vi "Periodic Tasks.vi"(8 "error in":errorcluster) -> ()   [LabVIEW 2015]
doc: "This VI runs in parallel to other tasks. It can contain as many user-defined periodic loops as you need. These can carry out PID or other sorts of timed response."
uses:
  Controls/ShooterState.ctl
  <vilib>/Rock Robotics/WPI/CAN/TalonSRX/WPI_CANTalonSRX_APIControlMode.ctl
  <vilib>/Rock Robotics/WPI/CAN/TalonSRX/WPI_CANTalonSRX_APIFeedbackSelect.ctl
  <vilib>/Rock Robotics/WPI/Utilities/WPI_GetSetVariantRefNum.vi
  <vilib>/Rock Robotics/WPI/MotorControl/WPI_MotorControlOpenCANTalonSRX.vi
  <vilib>/Rock Robotics/Network Tables/NT Read Boolean.vi
  Robot Global Data.vi
  <vilib>/Rock Robotics/Network Tables/NT Write Boolean.vi
  <vilib>/Rock Robotics/Network Tables/NT Write Number.vi
  navX-MXP-LabVIEW/navX Library v2/navX Library v2.lvlib
panel:
  in  "High Shoot RPM":dbl=15000.0
  in  "Low Shoot RPM":dbl=5000.0
  in  "Intake Outtake RPM":dbl=2000.0
  in  "Shoot High":dbl(slide)=0.708955223880597 scale=0.0..1.0
  in  "Intake Outtake":dbl(slide)=0.208955223880597 scale=0.0..1.0
  in  "Shoot Low":dbl(slide)=0.43283582089552236 scale=0.0..1.0
  out "Actual Speed Chart":dbl(graph)
  out "Actual Speed":dbl(knob) scale=-20000.0..20000.0 scale format="%4d"
  in  "Test Speed":dbl(slide)=0.6712328767123288 scale=0.0..1.0
  in  "TEST Device #":u8=2
  in  "Throttle Ramp Rate (percent/s)":dbl=1.0
  out "Current Feedback":dbl(graph)
  in  "F":dbl(slide)=0.025 scale=0.0..1.0
  in  "D":dbl(slide)=13.3 scale=0.0..10.0
  in  "I":dbl(slide)=2.47 scale=0.0..5.0
  in  "P":dbl(slide)=0.1573 scale=0.0..20.0
  in  "Set Speed (RPM)":dbl(slide) scale=0.0..20000.0
  out "Shooter State":T1=enum."No Movement"
  in  "Outtake Button":i32=2
  in  "Low Shoot":i32=1
  in  "High Shoot Button":i32=3
  in  "Intake Button":i32
  in  "I":dbl=2.473
  in  "F":dbl=0.025
  in  "D":dbl=13.3
  in  "P":dbl=0.1573
  in  "Reverse Feedback Sensor":bool
  in  "Slave Device Number":u8=3
  in  "Encoder Codes Per Rev":u16=1024
  in  "Master Device Number":u8=2
  out "Actual Speed (RPM)":dbl(knob) scale=-20000.0..20000.0 scale format="%4d"
  out "Feedback Chart":dbl(graph)
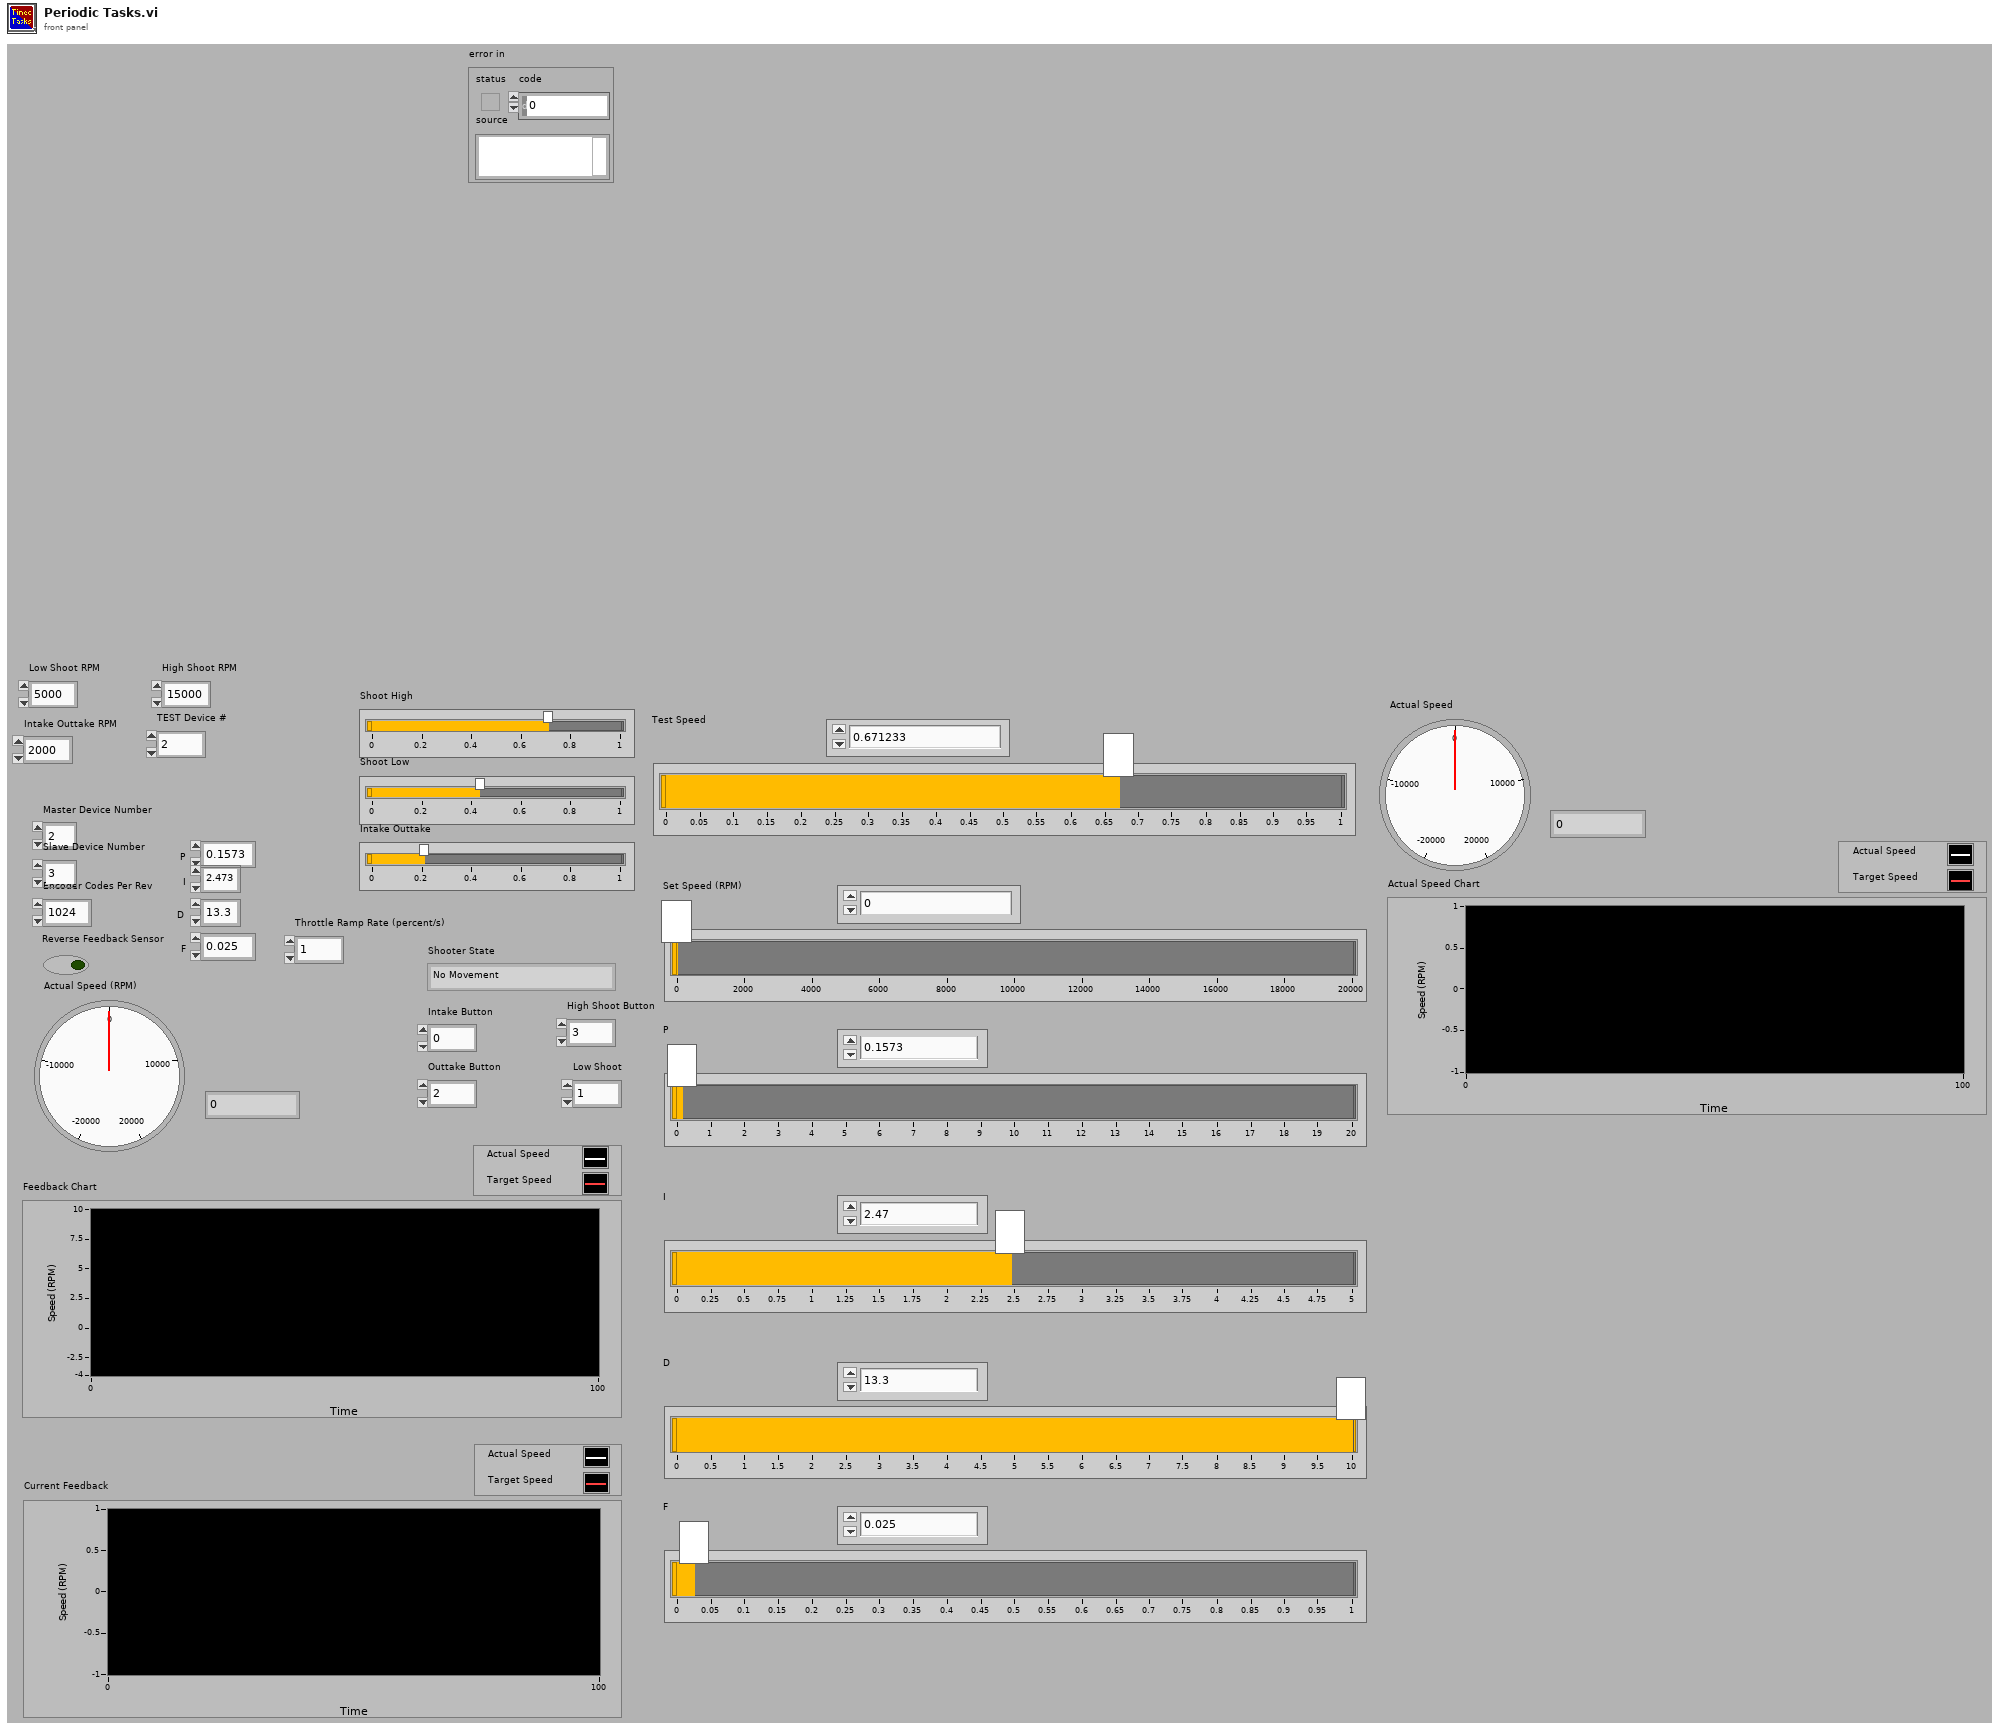
[diagram p1: front panel]
types:
  T1 = typedef "ShooterState.ctl" = enum16{"Test", "No Movement", "Intake", "Outtake", "Low Shoot", "High Shoot"}
  T2 = typedef "WPI_CANTalonSRX_APIControlMode.ctl" = enum8{"Percent VBus", "Speed", "Position", "Slave", "Unchanged / Invalid", "Voltage Compensation", "Current", "Motion Profile"}
  T3 = typedef "WPI_CANTalonSRX_APIFeedbackSelect.ctl" = enum16{"Digital Quadrature Encoder", "Analog Potentiometer", "Analog Encoder", "Count on Quad-A (Rising-Edge)", "Count on Quad-A (Falling-Edge)", "CTR Magnetic Enc (Absolute)", "CTR Magnetic Enc (Relative)", "Pulse Width"}
  T4 = typedef "WPI_MotorControlDeviceRef.ctl" = cluster{"DeviceStatus":errorcluster, "Type":T5, "PWM":cluster{"PWM Channel":T6, "DeadBand":T7}, "CAN":cluster{"Device Number":u8, "Control Mode":T8, "Semaphore":T9, "Max Vout":dbl, "TalonSRX Control Mode":T2}, "Invert":bool}
  T5 = typedef "WPI_MotorControlType.ctl" = enum16{"PWM", "CAN", "CANTalonSRX"}
  T6 = typedef "FPGA_DIOPWMChannel.ctl" = enum8{"PWM 0", "PWM 1", "PWM 2", "PWM 3", "PWM 4", "PWM 5", "PWM 6", "PWM 7", "PWM 8", "PWM 9", "PWM MXP 0", "PWM MXP 1", "PWM MXP 2", "PWM MXP 3", "PWM MXP 4", "PWM MXP 5", "PWM MXP 6", "PWM MXP 7", "PWM MXP 8", "PWM MXP 9", "Invalid"}
  T7 = typedef "WPI_PWMDeadband.ctl" = cluster{"Name":string, "maxPositivePwm":i32, "minPositivePwm":i32, "centerPwm":i32, "maxNegativePwm":i32, "minNegativePwm":i32, "angularRange":u16}
  T8 = typedef "WPI_CANJaguar_ControlMode.ctl" = enum8{"Percent VBus", "Current", "Speed", "Position", "Voltage"}
  T9 = typedef "Semaphore RefNum" = refnum<k1>
  T10 = typedef "WPI_CANTalonSRX_GlobalStatus.ctl" = cluster{"Applied Throttle":dbl, "Module Enabled":bool, "CAN Error":errorcluster, "Closed Loop Error":dbl, "Forward Limit Switch Closed":bool, "Reverse Limit Switch Closed":bool, "Sensor Position":dbl, "Sensor Velocity":dbl, "Current":dbl, "Sticky Fault - Over Temp":bool, "Sticky Fault - Under Voltage":bool, "Sticky Fault - Forward Limit":bool, "Sticky Fault - Reverse Limit":bool, "Sticky Fault - Forward Soft Limit":bool, "Sticky Fault - Reverse Soft Limit":bool, "Brake is Enabled":bool, "Encoder Position":dbl, "Encoder Velocity":dbl, "Encoder Index Count":dbl, "Encoder A Pin State":bool, "Encoder B Pin State":bool, "Encoder Index Pin State":bool, "Analog In":dbl, "Analog In Velocity":dbl, "Temperature (C)":dbl, "Battery Voltage":dbl, "Control 5 Is Supported":bool, "Current Profile Slot Select":dbl, "Pos Div 8":bool, "Vel Div 4":bool, "Pulse Width Position":i32, "Pulse Width Velocity":i32, "Pulse Width Rise To Rise (us)":i32, "Pulse Width Rise To Fall (us)":i32, "Mot Prof Active Is Under Run":bool, "Mot Prof Active Has Under Run":bool, "Mot Prof Active Is Last":bool, "Mot Prof Active Velocity Only":bool, "Mot Prof Active Is Valid":bool, "Mot Prof Buffer Is Full":bool, "Mot Prof Active Profile Slot Select":i32, "Mot Prof NextID":i32, "Mot Prof Count":i32, "Mot Prof Active Velocity":dbl, "Mot Prof Active Position":dbl, "Mot Prof Output Enable":i32}
  T11 = typedef "WPI_JoystickDevRef.ctl" = cluster{"Device":T12}
  T12 = typedef "WPI_JoystickDeviceEnum.ctl" = enum16{"USB 0", "USB 1", "USB 2", "USB 3", "USB 4", "USB 5"}
  T13 = typedef "WPI_RobotDriveDevRef.ctl" = cluster{"DevStatus":errorcluster, "Motors[]":T4[], "Square Inputs":bool, "Max Output":dbl}
  T14 = cluster{"JoystickDevRef":T11, "RobotDriveDevRef":T13}
  T15 = typedef "navX Library v2.lvlib/Z900_navX_DeviceTypeDef.ctl" = cluster{"Interface":cluster{"Protocol":T16, "Update Rate (4Hz-60Hz)":u8, "navX Open TypeDef":variant}, "Notify Packet":refnum<notifier>, "Loop VI Refnum":refnum<vi>, "Ready to Close Occurrence Refnum":refnum<k4>}
  T16 = typedef "navX Library v2.lvlib/Z900_navX_ProtocolTypeDef.ctl" = enum16{"SERIAL", "I2C", "SPI"}
  T17 = cluster{"Yaw":dbl, "Roll":dbl, "Pitch":dbl, "Heading":dbl, "Fused Heading":dbl}
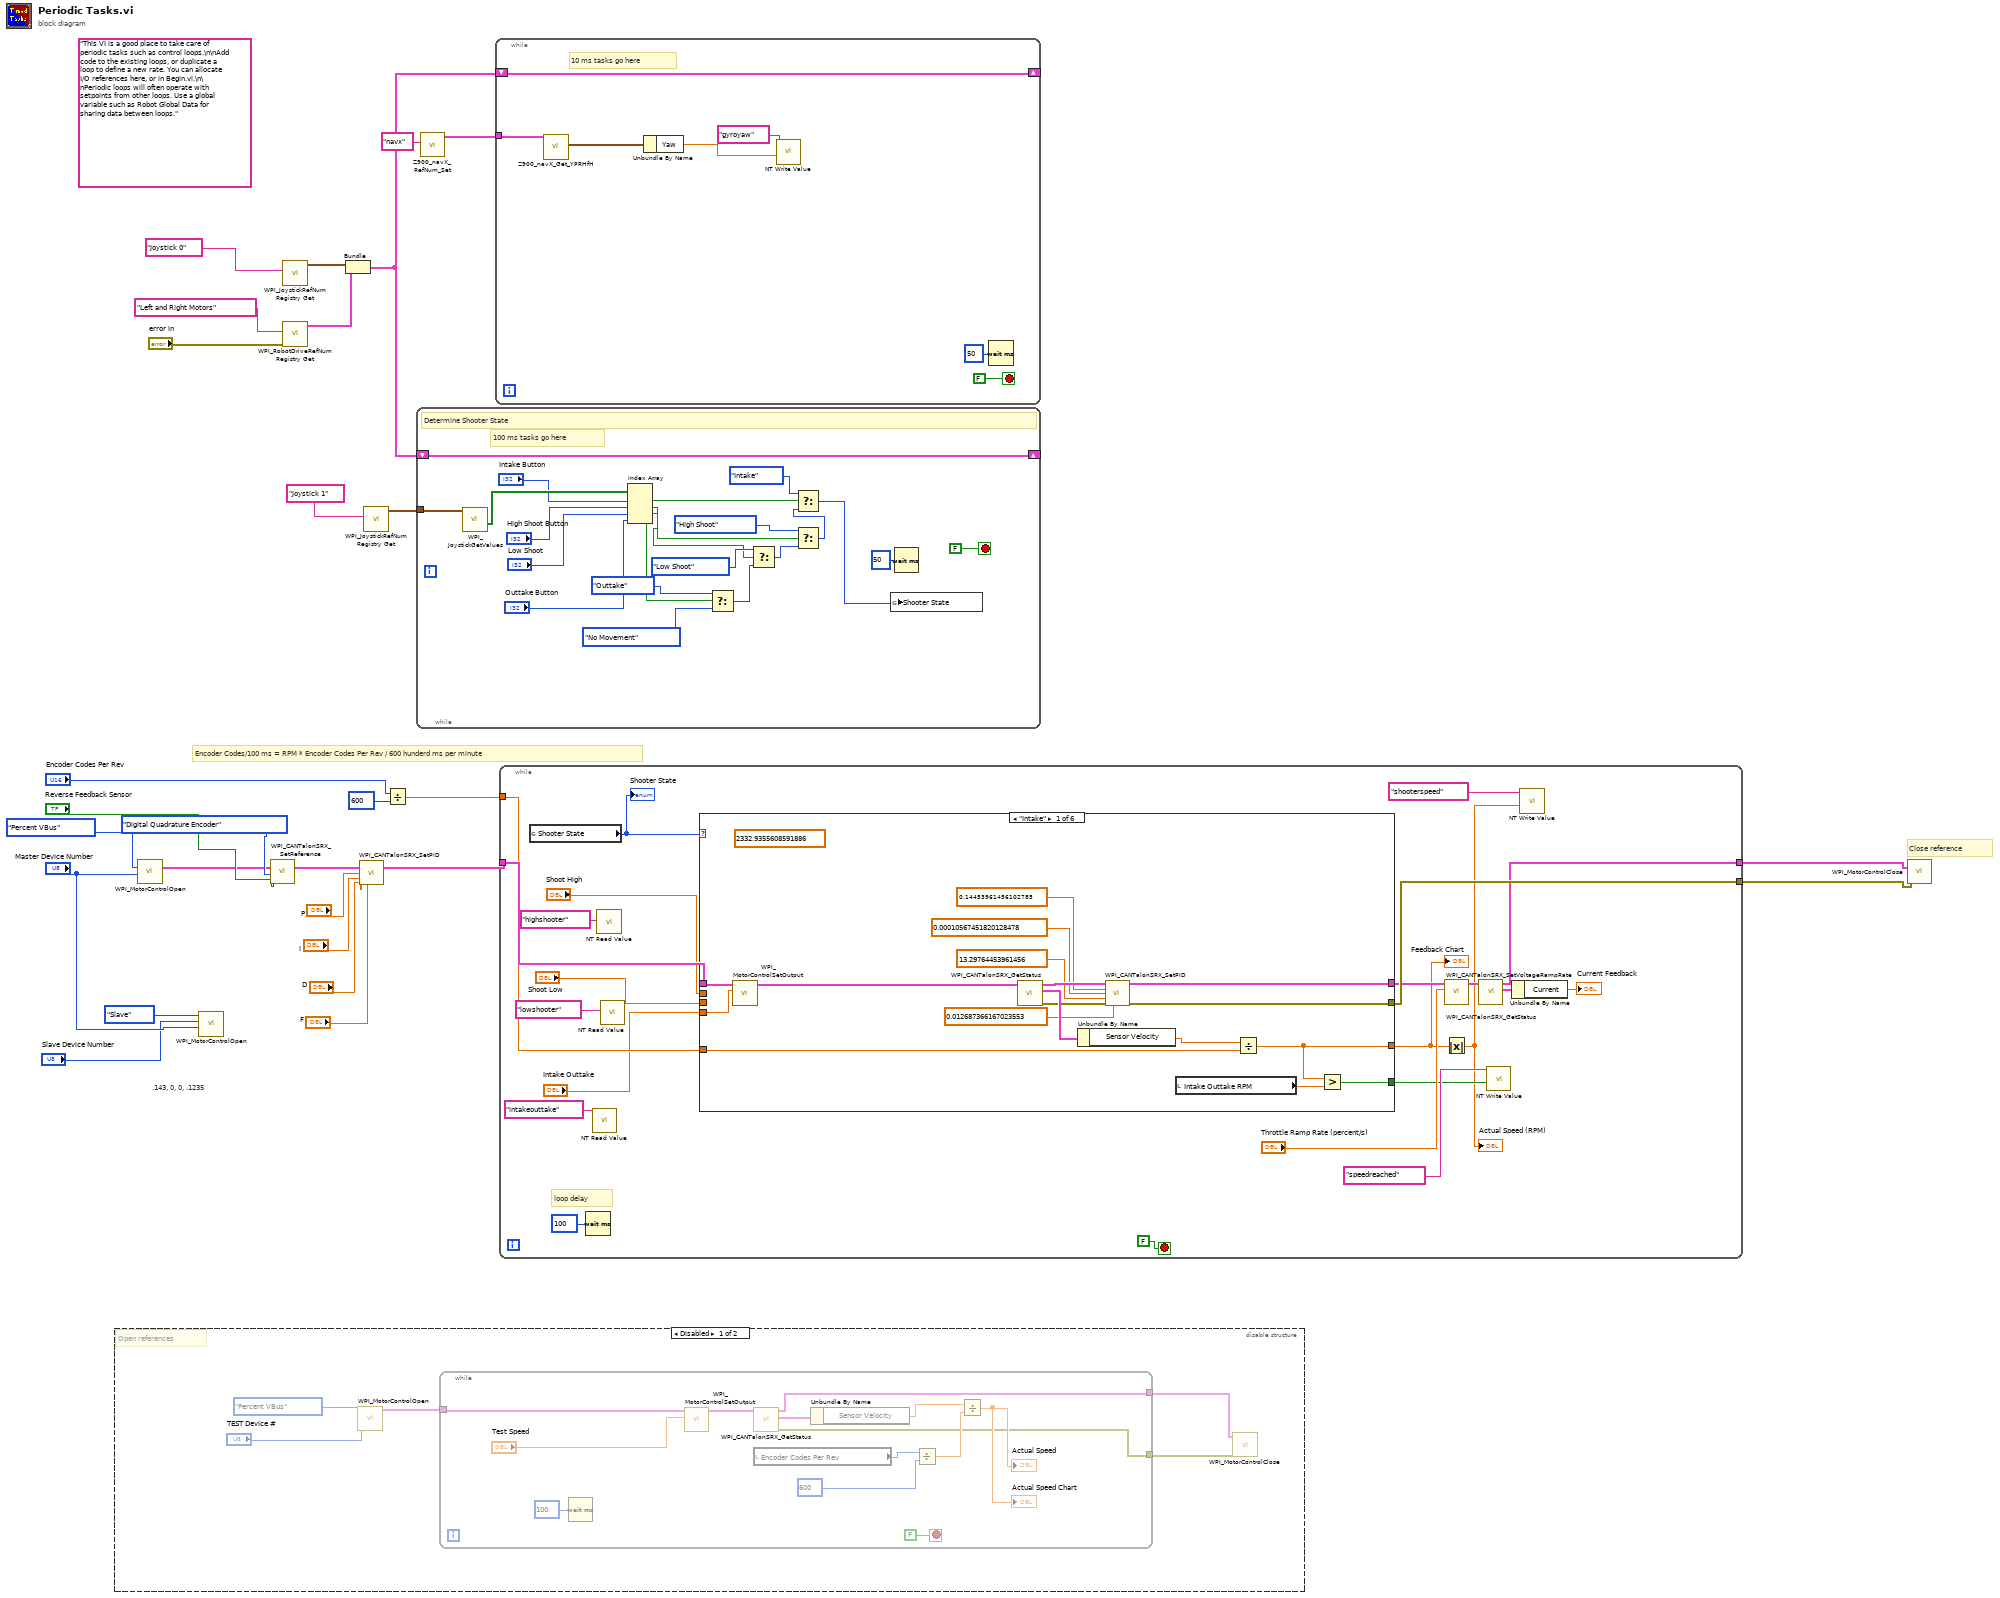
[diagram p0: block diagram]
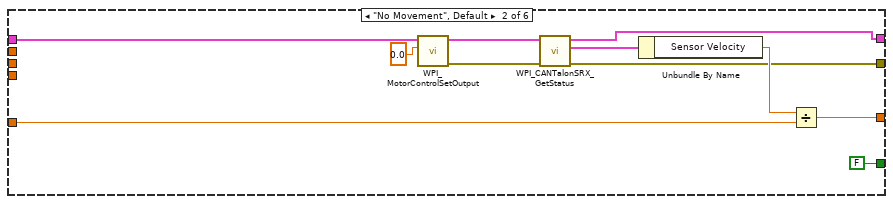
[diagram p3: hidden frame]
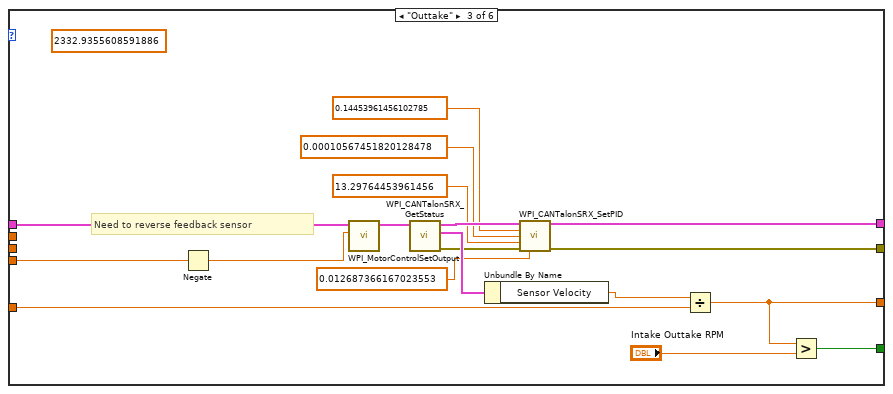
[diagram p4: hidden frame]
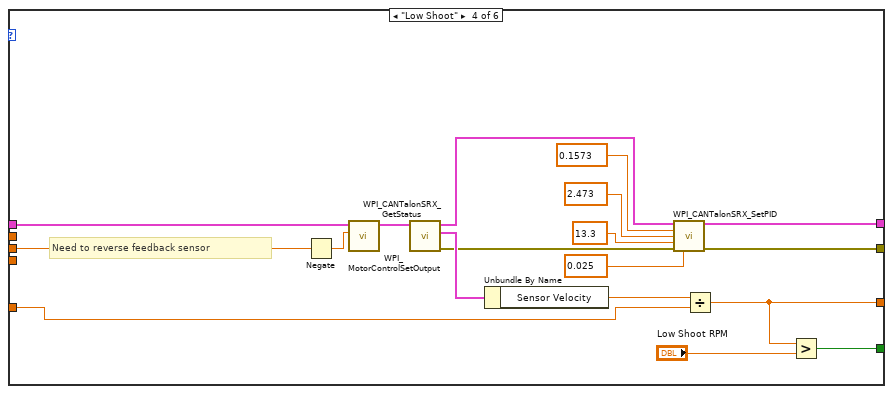
[diagram p5: hidden frame]
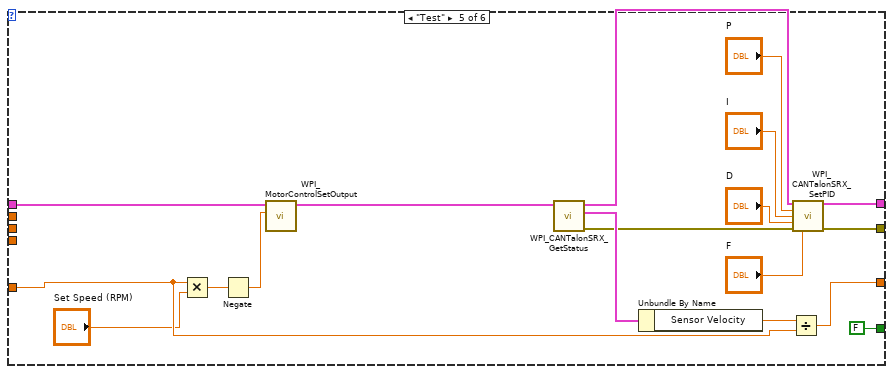
[diagram p6: hidden frame]
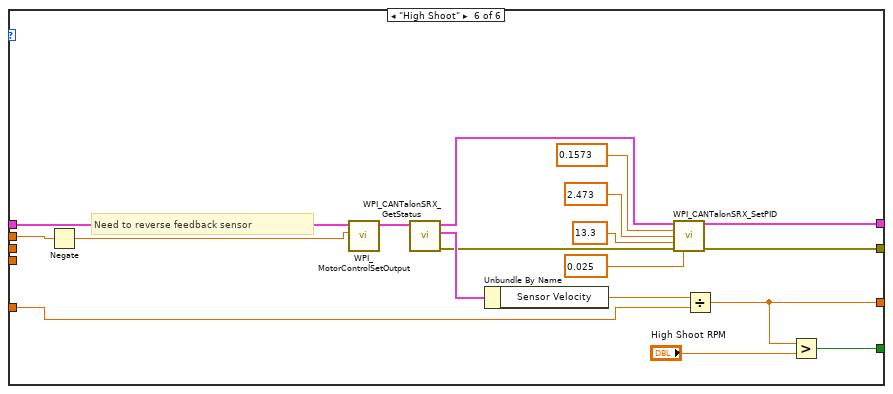
[diagram p7: hidden frame]
diagram:
  (unwired) "This VI is a good place to take care of periodic tasks such as control loops.\n\nAdd code to the existing loops, or duplicate a loop to define a new rate. You can allocate I/O references here, or in Begin.vi.\n\nPeriodic loops will often operate with setpoints from other loops. Use a global variable such as Robot Global Data for sharing data between loops."
  # ".143, 0, 0, .1235"
  # "Encoder Codes/100 ms = RPM * Encoder Codes Per Rev / 600 hunderd ms per minute"
  # "Close reference"
  n1 = disable-structure shown="Disabled" {
    frame Disabled {
      # "Open references"
      n2 = call-poly <vilib>:"WPI_MotorControlOpen.vi"("Device Number"="TEST Device #", "Control Mode"=WPI_CANTalonSRX_APIControlMode."Percent VBus") -> ("MotorControlDeviceRef"=w31:T4)  [unwired: 3 in, 6 out]
      n3 = while {
        tunnel: w31 -> [w44]
        tunnel: [w35] -> w30
        tunnel: [w34] -> w29
        stop <- FALSE stop-if-true
        n4 = Wait (ms)(milliseconds to wait=u32 100) -> ()  [unwired: 1 out]
        n5 = call <vilib>:"WPI_MotorControlSetOutput.vi"("Output"="Test Speed", "MotorControlDevRef"=w44) -> ("MotorControlDevRef"=w43:T4)  [unwired: 7 in, 2 out]
        n6 = local read "Encoder Codes Per Rev"() -> (w40:u16)
        n7 = call <vilib>:"WPI_CANTalonSRX_GetStatus.vi"("CAN Talon SRX Ref"=w43) -> ("error out"=w34:errorcluster, "Talon SRX Status"=w41:T10, "CAN Talon SRX Ref"=w35:T4)  [unwired: 8 in]
        n8 = Unbundle By Name(w41) -> ("Sensor Velocity"=w38:dbl)
        n9 = Divide(x=w40, y=u16 600) -> (x/y=w37:dbl)
        n10 = Divide(x=w38, y=w37) -> (x/y=→"Actual Speed" →"Actual Speed Chart":dbl)
      }
      n11 = call <vilib>:"WPI_MotorControlClose.vi"("error in (no error)"=w29, "MotorControlDevRef"=w30) -> ()  [unwired: 9 in, 1 out]
    }
    frame Enabled {
    }
  }
  n12 = call-poly <vilib>:"WPI_MotorControlOpen.vi"("Device Number"="Master Device Number", "Control Mode"=WPI_CANTalonSRX_APIControlMode."Percent VBus") -> ("MotorControlDeviceRef"=w10:T4)  [unwired: 3 in, 6 out]
  n13 = call-poly <vilib>:"WPI_MotorControlOpen.vi"("Master Device Number"="Master Device Number", "Device Number"="Slave Device Number", "Control Mode"=WPI_CANTalonSRX_APIControlMode."Slave") -> ()  [unwired: 2 in, 7 out]
  n14 = call <vilib>:"WPI_CANTalonSRX_SetReference.vi"("Reverse Feedback Sensor"="Reverse Feedback Sensor", "Feedback Reference"=WPI_CANTalonSRX_APIFeedbackSelect."Digital Quadrature Encoder", "CAN Talon SRX Ref"=w10) -> ("CAN Talon SRX Ref"=w9:T4)  [unwired: 7 in, 1 out]
  n15 = call <vilib>:"WPI_JoystickRefNum Registry Get.vi"("refnum name"="Joystick 0") -> ("JoystickDevRef"=w24:T11)  [unwired: 1 in, 9 out]
  n16 = call <vilib>:"WPI_RobotDriveRefNum Registry Get.vi"("error in (no error)"="error in", "refnum name"="Left and Right Motors") -> ("RobotDriveDevRef"=w26:T13)  [unwired: 9 out]
  n17 = Bundle("JoystickDevRef"=w24, "RobotDriveDevRef"=w26) -> (w25:T14)  [unwired: 1 out]
  n18 = call <vilib>:"WPI_CANTalonSRX_SetPID.vi"("CAN Talon SRX Ref"=w9, "P"="P", "I"="I", "D"="D", "F"="F") -> ("CAN Talon SRX Ref"=w22:T4)  [unwired: 9 in, 1 out]
  n19 = call <vilib>:"WPI_JoystickRefNum Registry Get.vi"("refnum name"="Joystick 1") -> ("JoystickDevRef"=w3:T11)  [unwired: 1 in, 9 out]
  n20 = Divide(x="Encoder Codes Per Rev", y=u16 600) -> (x/y=w18:dbl)
  n21 = while {
    shift-right: [w66] -> _
    shift-left: w25 -> [w66]
    tunnel: w3 -> [w65]
    stop <- FALSE stop-if-true
    # "100 ms tasks go here"
    # "Determine Shooter State"
    n22 = call <vilib>:"WPI_JoystickGetValues.vi"("JoystickDevRef"=w65) -> ("Buttons"=w64:bool[])  [unwired: 6 in, 4 out]
    n23 = Index Array(array=w64, index #1="Intake Button", index #2="High Shoot Button", index #3="Low Shoot", index #4="Outtake Button") -> (element #1=w60:bool, element #2=w58:bool, element #3=w52:bool, element #4=w51:bool)
    n24 = Select(t=ShooterState."Outtake", s=w51, f=ShooterState."No Movement") -> (s? t:f=w48:T1)
    n25 = Select(t=ShooterState."Low Shoot", s=w52, f=w48) -> (s? t:f=w53:T1)
    n26 = Select(t=ShooterState."High Shoot", s=w58, f=w53) -> (s? t:f=w56:T1)
    n27 = Select(t=ShooterState."Intake", s=w60, f=w56) -> (s? t:f=w47:T1)
    n28 = global write "Robot Global Data.vi" "Shooter State"(w47) -> ()
    n29 = Wait (ms)(milliseconds to wait=u32 50) -> ()  [unwired: 1 out]
  }
  n30 = call "Z900_navX_RefNum_Set.vi"("refnum name"="navx") -> ("navX Device"=w1:T15)  [unwired: 9 in, 1 out]
  n31 = while {
    shift-right: [w73] -> _
    shift-left: w25 -> [w73]
    tunnel: w1 -> [w72]
    stop <- FALSE stop-if-true
    # "10 ms tasks go here"
    n32 = call "Z900_navX_Get_YPRHfH.vi"("navX Device"=w72) -> ("YRPHfH"=w71:T17)  [unwired: 7 in, 3 out]
    n33 = Unbundle By Name(w71) -> ("Yaw"=w70:dbl)
    n34 = call-poly <vilib>:"NT Write Value.vi"("Numeric"=w70, "Name"="gyroyaw") -> ()  [unwired: 9 in, 1 out]
    n35 = Wait (ms)(milliseconds to wait=u32 50) -> ()  [unwired: 1 out]
  }
  n36 = while {
    tunnel: w22 -> [w97]
    tunnel: w18 -> [w96]
    tunnel: [w92] -> w5
    tunnel: [w95] -> w4
    stop <- FALSE stop-if-true
    # "loop delay"
    n37 = global read "Robot Global Data.vi" "Shooter State"() -> (w93:T1)
    "Shooter State" <- w93
    n38 = Wait (ms)(milliseconds to wait=u32 100) -> ()  [unwired: 1 out]
    n39 = call-poly <vilib>:"NT Read Value.vi"("Name"="intakeouttake") -> ()  [unwired: 9 in, 2 out]
    n40 = call-poly <vilib>:"NT Read Value.vi"("Name"="highshooter") -> ()  [unwired: 9 in, 2 out]
    n41 = call-poly <vilib>:"NT Read Value.vi"("Name"="lowshooter") -> ()  [unwired: 9 in, 2 out]
    n42 = case shown="\"Intake\"" w93 {
      tunnel: w97 -> [w115 w126 w144 w162 w180 w198]
      tunnel: w96 -> [w114 w125 w143 w161 w179 w197]
      tunnel: [w100 w121 w127 w145 w174 w182] -> w80
      tunnel: [w109 w120 w138 w156 w172 w192] -> w89
      tunnel: [w108 w119 w137 w155 w171 w191] -> w95
      tunnel: "Intake Outtake" -> [w102 _ w129 _ _ _]
      tunnel: "Shoot High" -> [_ _ _ _ _ w184]
      tunnel: "Shoot Low" -> [_ _ _ w146 _ _]
      tunnel: [w99 FALSE w130 w147 FALSE w181] -> w81
      frame "Intake" {
        (unwired) 2332.9355608591886 ("Set Speed (RPM)")
        n43 = call <vilib>:"WPI_MotorControlSetOutput.vi"("Output"=w102, "MotorControlDevRef"=w115) -> ("MotorControlDevRef"=w113:T4)  [unwired: 7 in, 2 out]
        n44 = call <vilib>:"WPI_CANTalonSRX_GetStatus.vi"("CAN Talon SRX Ref"=w113) -> ("error out"=w107:errorcluster, "Talon SRX Status"=w112:T10, "CAN Talon SRX Ref"=w110:T4)  [unwired: 8 in]
        n45 = Unbundle By Name(w112) -> ("Sensor Velocity"=w111:dbl)
        n46 = call <vilib>:"WPI_CANTalonSRX_SetPID.vi"("CAN Talon SRX Ref"=w110, "P"=0.14453961456102785 ("P 2"), "I"=0.00010567451820128478 ("P 3"), "D"=13.29764453961456 ("P 4"), "error in (no error)"=w107, "F"=0.012687366167023553 ("P 5")) -> ("CAN Talon SRX Ref"=w109:T4, "error out"=w108:errorcluster)  [unwired: 8 in]
        n47 = local read "Intake Outtake RPM"() -> (w101:dbl)
        n48 = Divide(x=w111, y=w114) -> (x/y=w100:dbl)
        n49 = Greater?(x=w100, y=w101) -> (0:w99:bool)
      }
      frame "No Movement", Default {
        n50 = call <vilib>:"WPI_MotorControlSetOutput.vi"("Output"=0.0, "MotorControlDevRef"=w126) -> ("error out"=w118:errorcluster, "MotorControlDevRef"=w124:T4)  [unwired: 7 in, 1 out]
        n51 = call <vilib>:"WPI_CANTalonSRX_GetStatus.vi"("error in (no error)"=w118, "CAN Talon SRX Ref"=w124) -> ("error out"=w119:errorcluster, "Talon SRX Status"=w123:T10, "CAN Talon SRX Ref"=w120:T4)  [unwired: 7 in]
        n52 = Unbundle By Name(w123) -> ("Sensor Velocity"=w122:dbl)
        n53 = Divide(x=w122, y=w125) -> (x/y=w121:dbl)
      }
      frame "Outtake" {
        (unwired) 2332.9355608591886 ("Set Speed (RPM)")
        # "Need to reverse feedback sensor"
        n54 = Negate(x=w129) -> (-x=w131:dbl)
        n55 = call <vilib>:"WPI_MotorControlSetOutput.vi"("Output"=w131, "MotorControlDevRef"=w144) -> ("MotorControlDevRef"=w142:T4)  [unwired: 7 in, 2 out]
        n56 = call <vilib>:"WPI_CANTalonSRX_GetStatus.vi"("CAN Talon SRX Ref"=w142) -> ("error out"=w136:errorcluster, "Talon SRX Status"=w141:T10, "CAN Talon SRX Ref"=w139:T4)  [unwired: 8 in]
        n57 = Unbundle By Name(w141) -> ("Sensor Velocity"=w140:dbl)
        n58 = call <vilib>:"WPI_CANTalonSRX_SetPID.vi"("CAN Talon SRX Ref"=w139, "P"=0.14453961456102785 ("P 2"), "I"=0.00010567451820128478 ("P 3"), "D"=13.29764453961456 ("P 4"), "error in (no error)"=w136, "F"=0.012687366167023553 ("P 5")) -> ("CAN Talon SRX Ref"=w138:T4, "error out"=w137:errorcluster)  [unwired: 8 in]
        n59 = Divide(x=w140, y=w143) -> (x/y=w127:dbl)
        n60 = Greater?(x=w127, y="Intake Outtake RPM") -> (0:w130:bool)
      }
      frame "Low Shoot" {
        # "Need to reverse feedback sensor"
        n61 = Negate(x=w146) -> (-x=w149:dbl)
        n62 = call <vilib>:"WPI_MotorControlSetOutput.vi"("Output"=w149, "MotorControlDevRef"=w162) -> ("MotorControlDevRef"=w160:T4)  [unwired: 7 in, 2 out]
        n63 = call <vilib>:"WPI_CANTalonSRX_GetStatus.vi"("CAN Talon SRX Ref"=w160) -> ("error out"=w154:errorcluster, "Talon SRX Status"=w159:T10, "CAN Talon SRX Ref"=w157:T4)  [unwired: 8 in]
        n64 = Unbundle By Name(w159) -> ("Sensor Velocity"=w158:dbl)
        n65 = call <vilib>:"WPI_CANTalonSRX_SetPID.vi"("CAN Talon SRX Ref"=w157, "P"=0.1573 ("P 2"), "I"=2.473 ("P 3"), "D"=13.3 ("P 4"), "error in (no error)"=w154, "F"=0.025 ("P 5")) -> ("CAN Talon SRX Ref"=w156:T4, "error out"=w155:errorcluster)  [unwired: 8 in]
        n66 = Divide(x=w158, y=w161) -> (x/y=w145:dbl)
        n67 = Greater?(x=w145, y="Low Shoot RPM") -> (0:w147:bool)
      }
      frame "Test" {
        n68 = Multiply(x=w179, y="Set Speed (RPM)") -> (x*y=w175:dbl)
        n69 = Negate(x=w175) -> (-x=w168:dbl)
        n70 = call <vilib>:"WPI_MotorControlSetOutput.vi"("Output"=w168, "MotorControlDevRef"=w180) -> ("MotorControlDevRef"=w178:T4)  [unwired: 7 in, 2 out]
        n71 = call <vilib>:"WPI_CANTalonSRX_GetStatus.vi"("CAN Talon SRX Ref"=w178) -> ("error out"=w170:errorcluster, "Talon SRX Status"=w177:T10, "CAN Talon SRX Ref"=w173:T4)  [unwired: 8 in]
        n72 = Unbundle By Name(w177) -> ("Sensor Velocity"=w176:dbl)
        n73 = Divide(x=w176, y=w179) -> (x/y=w174:dbl)
        n74 = call <vilib>:"WPI_CANTalonSRX_SetPID.vi"("CAN Talon SRX Ref"=w173, "P"="P", "I"="I", "D"="D", "error in (no error)"=w170, "F"="F") -> ("CAN Talon SRX Ref"=w172:T4, "error out"=w171:errorcluster)  [unwired: 8 in]
      }
      frame "High Shoot" {
        # "Need to reverse feedback sensor"
        n75 = Negate(x=w184) -> (-x=w185:dbl)
        n76 = call <vilib>:"WPI_MotorControlSetOutput.vi"("Output"=w185, "MotorControlDevRef"=w198) -> ("MotorControlDevRef"=w196:T4)  [unwired: 7 in, 2 out]
        n77 = call <vilib>:"WPI_CANTalonSRX_GetStatus.vi"("CAN Talon SRX Ref"=w196) -> ("error out"=w190:errorcluster, "Talon SRX Status"=w195:T10, "CAN Talon SRX Ref"=w193:T4)  [unwired: 8 in]
        n78 = Unbundle By Name(w195) -> ("Sensor Velocity"=w194:dbl)
        n79 = call <vilib>:"WPI_CANTalonSRX_SetPID.vi"("CAN Talon SRX Ref"=w193, "P"=0.1573 ("P 2"), "I"=2.473 ("P 3"), "D"=13.3 ("P 4"), "error in (no error)"=w190, "F"=0.025 ("P 5")) -> ("CAN Talon SRX Ref"=w192:T4, "error out"=w191:errorcluster)  [unwired: 8 in]
        n80 = Divide(x=w194, y=w197) -> (x/y=w182:dbl)
        n81 = Greater?(x=w182, y="High Shoot RPM") -> (0:w181:bool)
      }
    }
    "Feedback Chart" <- w80
    n82 = call <vilib>:"WPI_CANTalonSRX_SetVoltageRampRate.vi"("Throttle Ramp Rate (percent/s)"="Throttle Ramp Rate (percent/s)", "CAN Talon SRX Ref"=w89) -> ("CAN Talon SRX Ref"=w88:T4)  [unwired: 8 in, 1 out]
    n83 = Absolute Value(x=w80) -> (abs(x)=w79:dbl)
    "Actual Speed (RPM)" <- w79
    n84 = call <vilib>:"WPI_CANTalonSRX_GetStatus.vi"("CAN Talon SRX Ref"=w88) -> ("Talon SRX Status"=w91:T10, "CAN Talon SRX Ref"=w92:T4)  [unwired: 8 in, 1 out]
    n85 = call-poly <vilib>:"NT Write Value.vi"("Boolean"=w81, "Name"="speedreached") -> ()  [unwired: 9 in, 1 out]
    n86 = Unbundle By Name(w91) -> ("Current"=→"Current Feedback":dbl)
    n87 = call-poly <vilib>:"NT Write Value.vi"("Numeric"=w79, "Name"="shooterspeed") -> ()  [unwired: 9 in, 1 out]
  }
  n88 = call <vilib>:"WPI_MotorControlClose.vi"("error in (no error)"=w4, "MotorControlDevRef"=w5) -> ()  [unwired: 9 in, 1 out]
